vi "EnviarParametros_global.vi"(0 "VISA resource name":refnum<visa-resource-name>, 1 "Cluster":T1 {"MODOS"."Ring" items=["TEST ASICS"=1, "TRASPASO ASICS"=2, "MOVER CABEZAL"=3, "CALIBRACION"=4]}, 5 "error in (no error)":errorcluster) -> (14 "VISA resource name 2":refnum<visa-resource-name>, 17 "read buffer":string, 18 "enviados":string, 19 "error IO":errorcluster)   [LabVIEW 2019]
uses:
  Data_to_Arduino.ctl
  <vilib>/Utility/error.llb/Error Cluster From Error Code.vi
  <vilib>/ErrorRing/Error Ring.xnode
panel:
  out "return count 2":u32
  out "return count":u32
  out "Parametros enviados = Parametros leídos?":bool
  # "/* Teoricamente:\n1mm= 91 pasos\n1cm = 910 pasos\n10 cm = 9100 pasos\n0.1 mm = 9 pasos aprox\n*/"
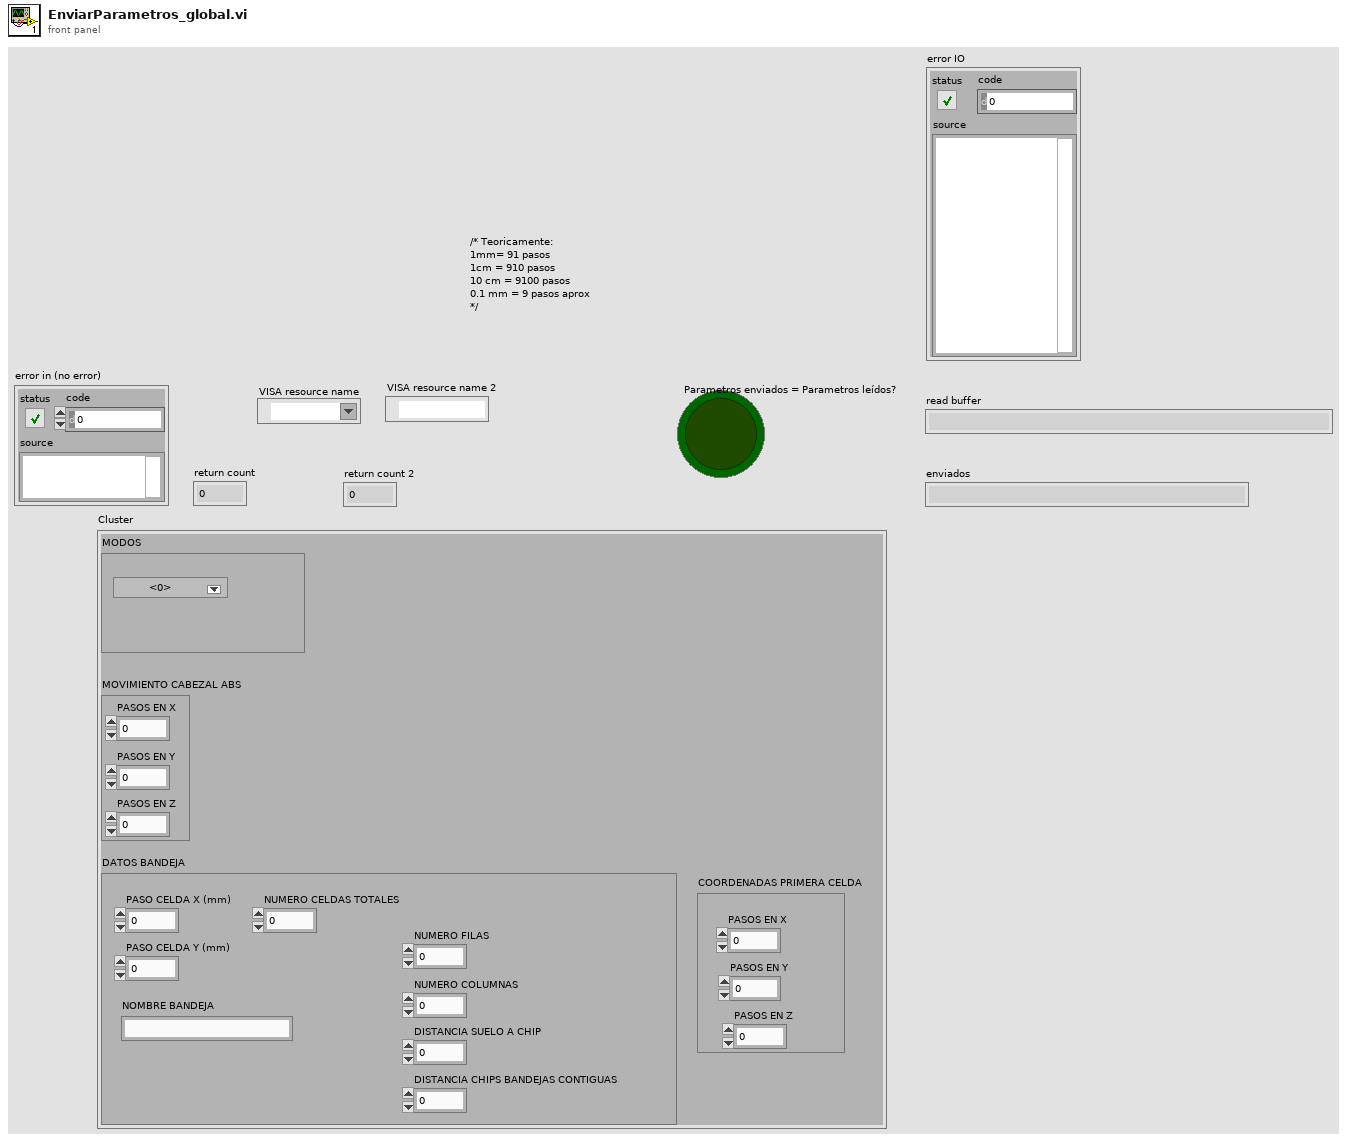
[diagram p1: front panel]
types:
  T1 = typedef "Data_to_Arduino.ctl" = cluster{"MODOS":cluster{"Ring":u16}, "MOVIMIENTO CABEZAL ABS":cluster{"PASOS EN X":i32, "PASOS EN Y":i32, "PASOS EN Z":i32}, "DATOS BANDEJA":cluster{"PASO CELDA X (mm)":dbl, "PASO CELDA Y (mm)":dbl, "NOMBRE BANDEJA":string, "NUMERO COLUMNAS":u16, "NUMERO FILAS":u16, "NUMERO CELDAS TOTALES":u16, "DISTANCIA SUELO A CHIP":dbl, "DISTANCIA CHIPS BANDEJAS CONTIGUAS":dbl}, "COORDENADAS PRIMERA CELDA":cluster{"PASOS EN X":dbl, "PASOS EN Y":dbl, "PASOS EN Z":dbl}}
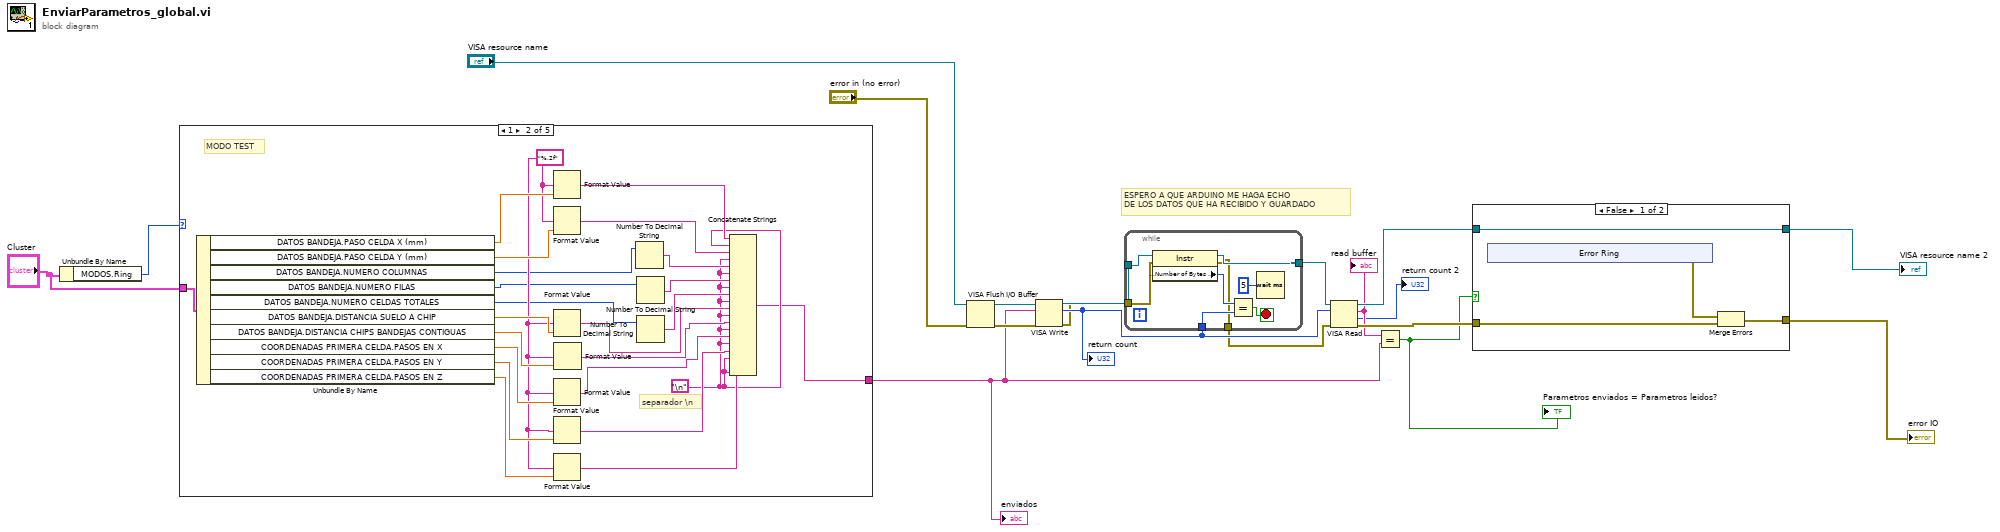
[diagram p0: block diagram]
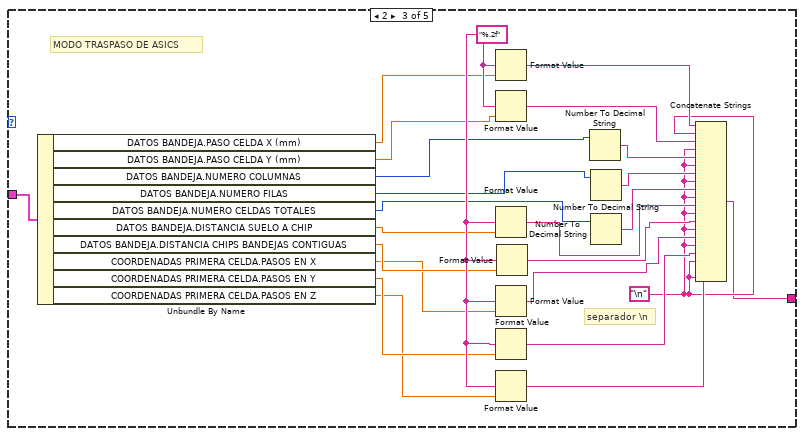
[diagram p3: hidden frame]
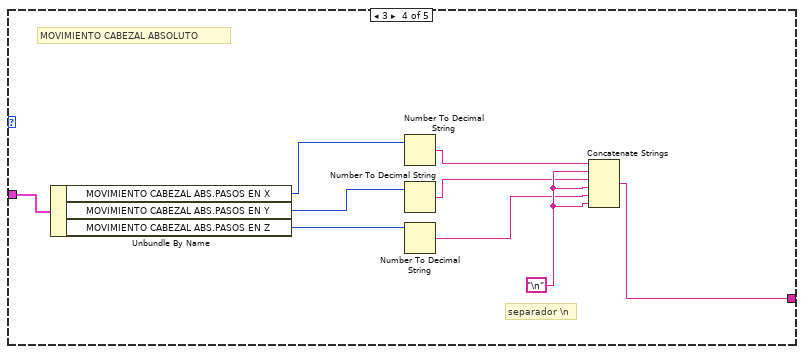
[diagram p4: hidden frame]
diagram:
  # "ESPERO A QUE ARDUINO ME HAGA ECHO\nDE LOS DATOS QUE HA RECIBIDO Y GUARDADO"
  n1 = Unbundle By Name("Cluster") -> ("MODOS.Ring"=w3:u16)
  n2 = case shown="1" w3 {
    tunnel: "Cluster" -> [_ w43 w67 w76 _]
    tunnel: [_ w20 w47 w74 _] -> w1
    frame 0, Default {
    }
    frame 1 {
      w35 = "%.2f" ("format string")
      w21 = "\n"
      # "separador \\n"
      # "MODO TEST"
      n3 = Unbundle By Name(w43) -> ("DATOS BANDEJA.PASO CELDA X (mm)"=w42:dbl, "DATOS BANDEJA.PASO CELDA Y (mm)"=w41:dbl, "DATOS BANDEJA.NUMERO COLUMNAS"=w34:u16, "DATOS BANDEJA.NUMERO FILAS"=w33:u16, "DATOS BANDEJA.NUMERO CELDAS TOTALES"=w32:u16, "DATOS BANDEJA.DISTANCIA SUELO A CHIP"=w40:dbl, "DATOS BANDEJA.DISTANCIA CHIPS BANDEJAS CONTIGUAS"=w39:dbl, "COORDENADAS PRIMERA CELDA.PASOS EN X"=w38:dbl, "COORDENADAS PRIMERA CELDA.PASOS EN Y"=w37:dbl, "COORDENADAS PRIMERA CELDA.PASOS EN Z"=w36:dbl)
      n4 = Format Value(format string=w35, value (0)=w42) -> (output string=w31:string)  [unwired: 1 in]
      n5 = Format Value(format string=w35, value (0)=w41) -> (output string=w30:string)  [unwired: 1 in]
      n6 = Format Value(format string=w35, value (0)=w40) -> (output string=w26:string)  [unwired: 1 in]
      n7 = Format Value(format string=w35, value (0)=w38) -> (output string=w24:string)  [unwired: 1 in]
      n8 = Format Value(format string=w35, value (0)=w37) -> (output string=w23:string)  [unwired: 1 in]
      n9 = Format Value(format string=w35, value (0)=w36) -> (output string=w22:string)  [unwired: 1 in]
      n10 = Format Value(format string=w35, value (0)=w39) -> (output string=w25:string)  [unwired: 1 in]
      n11 = Number To Decimal String(number=w34) -> (decimal integer string=w29:string)  [unwired: 1 in]
      n12 = Number To Decimal String(number=w33) -> (decimal integer string=w28:string)  [unwired: 1 in]
      n13 = Number To Decimal String(number=w32) -> (decimal integer string=w27:string)  [unwired: 1 in]
      n14 = Concatenate Strings(w31, w21, w30, w21, w29, w21, w28, w21, w27, w21, w26, w21, w25, w21, w24, w21, w23, w21, w22, w21) -> (w20:string)
    }
    frame 2 {
      w66 = "%.2f" ("format string")
      w55 = "\n"
      # "separador \\n"
      # "MODO TRASPASO DE ASICS"
      n15 = Unbundle By Name(w67) -> ("DATOS BANDEJA.PASO CELDA X (mm)"=w54:dbl, "DATOS BANDEJA.PASO CELDA Y (mm)"=w53:dbl, "DATOS BANDEJA.NUMERO COLUMNAS"=w46:u16, "DATOS BANDEJA.NUMERO FILAS"=w45:u16, "DATOS BANDEJA.NUMERO CELDAS TOTALES"=w44:u16, "DATOS BANDEJA.DISTANCIA SUELO A CHIP"=w52:dbl, "DATOS BANDEJA.DISTANCIA CHIPS BANDEJAS CONTIGUAS"=w51:dbl, "COORDENADAS PRIMERA CELDA.PASOS EN X"=w50:dbl, "COORDENADAS PRIMERA CELDA.PASOS EN Y"=w49:dbl, "COORDENADAS PRIMERA CELDA.PASOS EN Z"=w48:dbl)
      n16 = Format Value(format string=w66, value (0)=w54) -> (output string=w65:string)  [unwired: 1 in]
      n17 = Format Value(format string=w66, value (0)=w53) -> (output string=w64:string)  [unwired: 1 in]
      n18 = Format Value(format string=w66, value (0)=w52) -> (output string=w60:string)  [unwired: 1 in]
      n19 = Format Value(format string=w66, value (0)=w50) -> (output string=w58:string)  [unwired: 1 in]
      n20 = Format Value(format string=w66, value (0)=w49) -> (output string=w57:string)  [unwired: 1 in]
      n21 = Format Value(format string=w66, value (0)=w48) -> (output string=w56:string)  [unwired: 1 in]
      n22 = Format Value(format string=w66, value (0)=w51) -> (output string=w59:string)  [unwired: 1 in]
      n23 = Number To Decimal String(number=w46) -> (decimal integer string=w63:string)  [unwired: 1 in]
      n24 = Number To Decimal String(number=w45) -> (decimal integer string=w62:string)  [unwired: 1 in]
      n25 = Number To Decimal String(number=w44) -> (decimal integer string=w61:string)  [unwired: 1 in]
      n26 = Concatenate Strings(w65, w55, w64, w55, w63, w55, w62, w55, w61, w55, w60, w55, w59, w55, w58, w55, w57, w55, w56, w55) -> (w47:string)
    }
    frame 3 {
      w75 = "\n"
      # "separador \\n"
      # "MOVIMIENTO CABEZAL ABSOLUTO"
      n27 = Unbundle By Name(w76) -> ("MOVIMIENTO CABEZAL ABS.PASOS EN X"=w73:i32, "MOVIMIENTO CABEZAL ABS.PASOS EN Y"=w71:i32, "MOVIMIENTO CABEZAL ABS.PASOS EN Z"=w69:i32)
      n28 = Number To Decimal String(number=w73) -> (decimal integer string=w72:string)  [unwired: 1 in]
      n29 = Number To Decimal String(number=w71) -> (decimal integer string=w70:string)  [unwired: 1 in]
      n30 = Number To Decimal String(number=w69) -> (decimal integer string=w68:string)  [unwired: 1 in]
      n31 = Concatenate Strings(w72, w75, w70, w75, w68, w75) -> (w74:string)
    }
    frame 4 {
      # "CALIBRACION"
    }
  }
  "enviados" <- w1
  n32 = VISA Flush I/O Buffer(VISA resource name="VISA resource name", error in (no error)="error in (no error)") -> (VISA resource name out=w10:refnum<visa-resource-name>, error out=w11:errorcluster)  [unwired: 1 in]
  n33 = VISA Write(VISA resource name=w10, write buffer=w1, error in (no error)=w11) -> (VISA resource name out=w7:refnum<visa-resource-name>, return count=w8:u32, error out=w5:errorcluster)
  "return count" <- w8
  n34 = while {
    tunnel: w8 -> [w83]
    tunnel: w7 -> [w81]
    tunnel: [w80] -> w6
    tunnel: w5 -> [w79]
    tunnel: [w78] -> w4
    stop <- w82 stop-if-true
    n35 = property class="Instr"(reference=w81, error in=w79) -> (reference out=w80:refnum<visa-resource-name>, error out=w78:errorcluster, "Serial Settings:Number of Bytes at Serial Port"=w84:u32)
    n36 = Equal?(x=w84, y=w83) -> (x = y?=w82:bool)
    n37 = Wait (ms)(milliseconds to wait=u32 5) -> ()  [unwired: 1 out]
  }
  n38 = VISA Read(VISA resource name=w6, byte count=w8, error in (no error)=w4) -> (VISA resource name out=w15:refnum<visa-resource-name>, read buffer=w12:string, return count=→"return count 2":u32, error out=w17:errorcluster)
  "read buffer" <- w12
  n39 = Equal?(x=w12, y=w1) -> (x = y?=w13:bool)
  "Parametros enviados = Parametros leídos?" <- w13
  n40 = case shown="False" w13 {
    tunnel: w17 -> [w87 w94]
    tunnel: [w86 w94] -> w16
    tunnel: w15 -> [w85 w95]
    tunnel: [w85 w95] -> w14
    frame False {
      n41 = xnode "Error Ring"() -> ("error out"=w88:errorcluster)
      n42 = Merge Errors(w88, w87) -> (w86:errorcluster)
    }
    frame True {
    }
  }
  "error IO" <- w16
  "VISA resource name 2" <- w14
